vi "tlc_Timing Module.vi"(7 "Timer Command":T1, 8 "error in (no error)":errorcluster, 10 "Target Time":u32) -> (0 "error out":errorcluster, 1 "Elapsed Time":dbl, 2 "Done?":bool)   [LabVIEW 2010]
doc: "This VI is a functional global variable that keeps track the amount of time elapsed since a Start command was sent to the VI."
uses:
  tlc_Timing Command Control.ctl
panel:
  # "Input"
  # "Output"
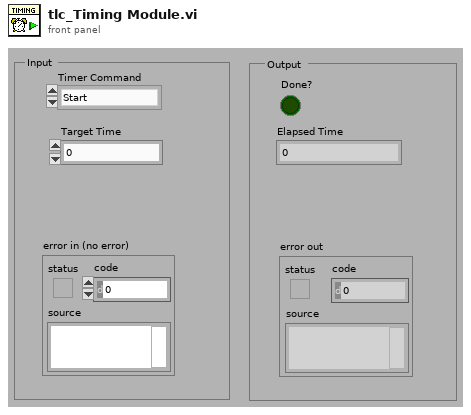
[diagram p1: front panel]
types:
  T1 = typedef "tlc_Timing Command Control.ctl" = enum16{"Start", "Check Time"}
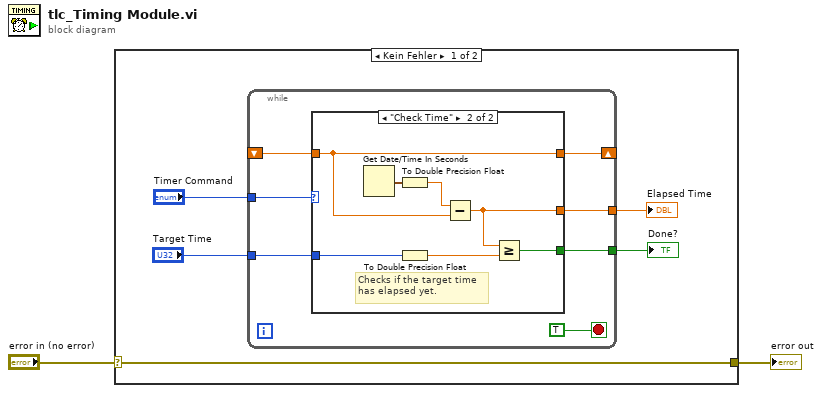
[diagram p0: block diagram]
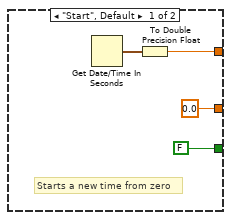
[diagram p2: hidden frame]
diagram:
  n1 = case shown="Kein Fehler" "error in (no error)" {
    selector: "error in (no error)" -> [w7 w26]
    tunnel: [w7 w26] -> w2
    frame No Error {
      n2 = while {
        tunnel: "Timer Command" -> [w14]
        shift-right: [w13] -> _
        shift-left: _ -> [w12]
        tunnel: [w11] -> w5
        tunnel: [w10] -> w4
        tunnel: "Target Time" -> [w9]
        stop <- TRUE stop-if-true
        n3 = case shown="\"Check Time\"" w14 {
          tunnel: [w17 w23] -> w13
          tunnel: w12 -> [_ w23]
          tunnel: [0.0 ("double precision float") w22] -> w11
          tunnel: [FALSE w19] -> w10
          tunnel: w9 -> [_ w20]
          frame "Start", Default {
            # "Starts a new time from zero"
            n4 = Get Date/Time In Seconds() -> (seconds since 1Jan1904=w18:timestamp)
            n5 = To Double Precision Float(number=w18) -> (double precision float=w17:dbl)
          }
          frame "Check Time" {
            # "Checks if the target time\nhas elapsed yet."
            n6 = Get Date/Time In Seconds() -> (seconds since 1Jan1904=w25:timestamp)
            n7 = To Double Precision Float(number=w25) -> (double precision float=w24:dbl)
            n8 = To Double Precision Float(number=w20) -> (double precision float=w21:dbl)
            n9 = Subtract(x=w24, y=w23) -> (x-y=w22:dbl)
            n10 = Greater Or Equal?(x=w22, y=w21) -> (x >= y?=w19:bool)
          }
        }
      }
      "Done?" <- w4
      "Elapsed Time" <- w5
    }
    frame Error {
      (unwired) u32 0 ("Update Rate")
    }
  }
  "error out" <- w2
